vi "Script_Timing_Extract_Excit_Acq.vi"(7 "Script Text":string="script PireneaGas2sExcitAcq8s\n   wait until scriptTrigger0 \n   wait dd\n   generate AutLaserOn\n   wait 49000\n   generate AutLaserOnFilterOff\n   wait 1000\n   wait 600\n   generate AutLaserOnFilterOffTrapStart\n   wait 300\n   generate AutLaserOnFilterOffTrapStop\n   wait 2000\n   generate AutLaserOnFilterOn\n   wait 47100\n   generate AutLaserOff\n   wait 1950000\n   generate Gas1On\n   wait 150000\n   generate Gas1Off\n   wait 5850000\n   generate ExcitAcq\n   wait 1000000\n   generate FilterOff\n   wait 1000\n   generate FilterOffEmptyingStart\n   wait 1000000\n   generate FilterOffEmptyingStop\n   wait 2000\n   generate Zeros\nend script", 8 "error in (no error)":errorcluster, 9 "Script File":string="PireneaFree4sExcitAcq5s.txt", 10 "Script Path":path=path "D:/PIRENEA/TIMING_SCRIPTS") -> (0 "error out":errorcluster, 2 "Number of Excits":i16, 3 "Number of Acqs":i16)   [LabVIEW 2018]
uses:
  Global_Variables.vi
  <vilib>/regexp/Match Regular Expression.xnode
panel:
  out "Table of Excit":string[](array[string])
  out "Table of Acq":string[](array[string])
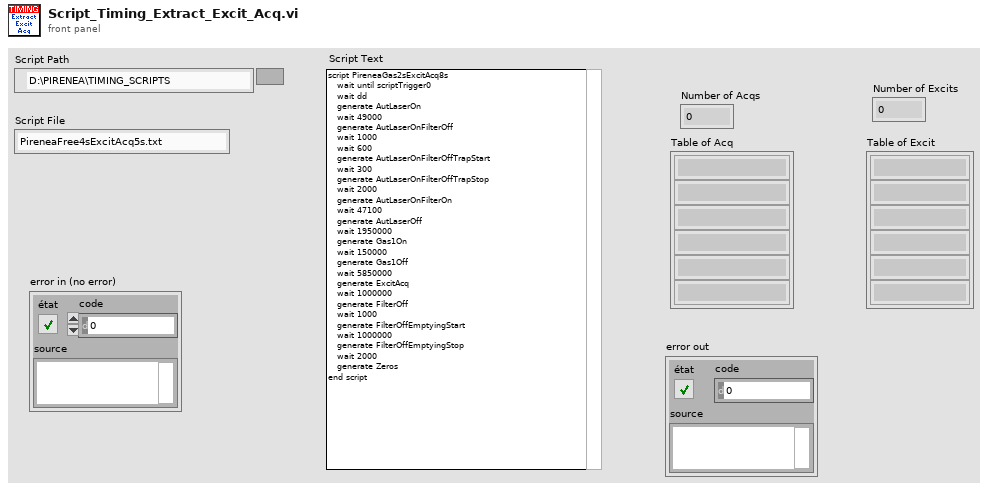
[diagram p1: front panel]
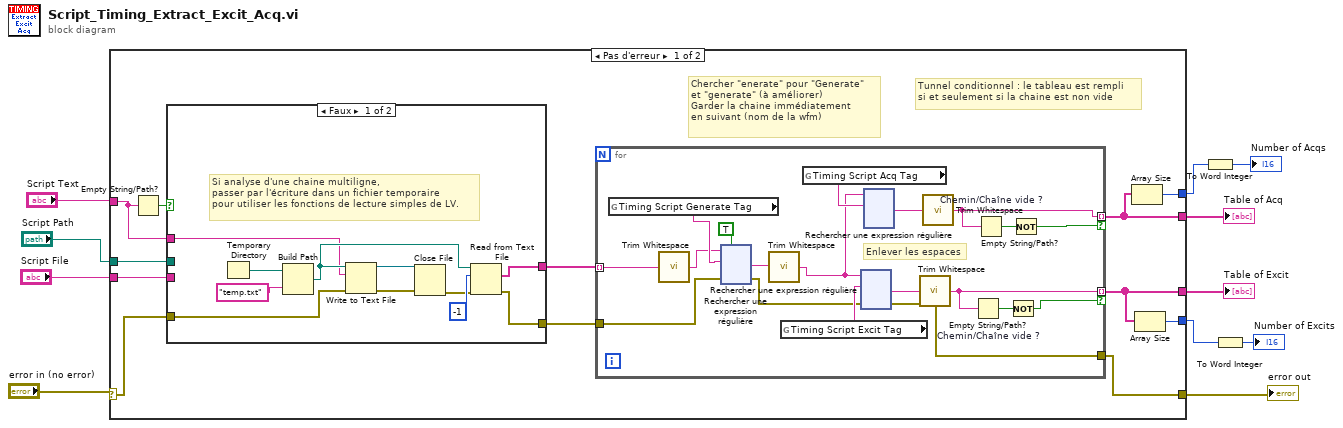
[diagram p0: block diagram]
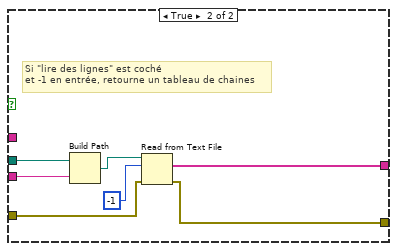
[diagram p2: hidden frame]
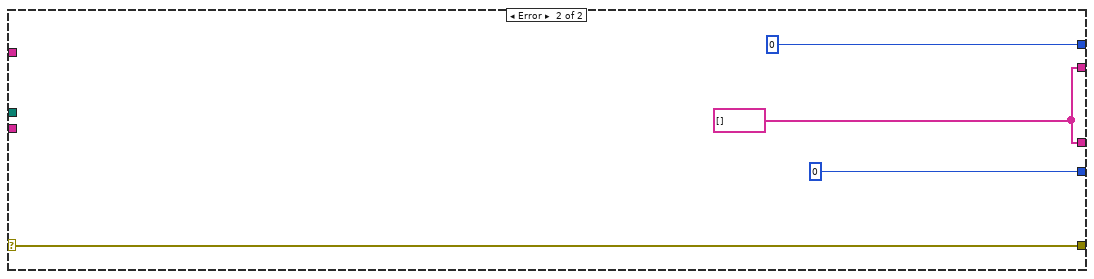
[diagram p3: hidden frame]
diagram:
  n1 = case shown="Pas d'erreur" "error in (no error)" {
    selector: "error in (no error)" -> [w14 w406]
    tunnel: "Script File" -> [w23 _]
    tunnel: [w12 w406] -> w9
    tunnel: "Script Path" -> [w22 _]
    tunnel: [w20 w405] -> w7
    tunnel: [w18 w405] -> w6
    tunnel: [w19 0] -> w5
    tunnel: [w17 0] -> w4
    tunnel: "Script Text" -> [w15 _]
    frame No Error {
      # "Tunnel conditionnel : le tableau est rempli\nsi et seulement si la chaine est non vide"
      # "Chercher \"enerate\" pour \"Generate\"\net \"generate\" (à améliorer)\nGarder la chaine immédiatement\nen suivant (nom de la wfm)"
      n2 = Empty String/Path?(string/path=w15) -> (empty?=w16:bool)
      n3 = case shown="Faux" w16 {
        tunnel: w23 -> [_ w41]
        tunnel: w22 -> [_ w40]
        tunnel: [w26 w37] -> w21
        tunnel: w15 -> [w27 _]
        tunnel: w14 -> [w25 w36]
        tunnel: [w24 w35] -> w13
        frame False {
          # "Si analyse d'une chaine multiligne,\npasser par l'écriture dans un fichier temporaire\npour utiliser les fonctions de lecture simples de LV."
          n4 = Temporary Directory() -> (w33:path)
          n5 = Build Path(base path=w33, name or relative path="temp.txt" ("nom ou chemin relatif")) -> (appended path=w30:path)
          n6 = Write to Text File(file (use dialog)=w30, text=w27, error in=w25) -> (refnum out=w31:refnum<file>, error out=w32:errorcluster)  [unwired: 1 in, 1 out]
          n7 = Close File(refnum=w31, error in=w32) -> (error out=w28:errorcluster)  [unwired: 1 out]
          n8 = Read from Text File(file (use dialog)=w30, count=-1 ("nombre"), error in=w28) -> (text=w26:string[], error out=w24:errorcluster)  [unwired: 1 in, 2 out]
        }
        frame True {
          # "Si \"lire des lignes\" est coché\net -1 en entrée, retourne un tableau de chaines"
          n9 = Build Path(base path=w40, name or relative path=w41) -> (appended path=w39:path)
          n10 = Read from Text File(file (use dialog)=w39, count=-1 ("nombre"), error in=w36) -> (text=w37:string[], error out=w35:errorcluster)  [unwired: 1 in, 2 out]
        }
      }
      n11 = for {
        tunnel: w21 -> [w60] mode=indexing
        tunnel: [w57] -> w20 mode=indexing if=w58
        tunnel: [w52] -> w18 mode=indexing if=w51
        tunnel: w13 -> [w45]
        tunnel: [w42] -> w12
        # "Enlever les espaces"
        n12 = global read "Global_Variables.vi" "Timing Script Generate Tag"() -> (w48:string)
        n13 = call <vilib>:"Trim Whitespace.vi"("string"=w60) -> ("trimmed string"=w47:string)  [unwired: 1 in]
        n14 = xnode "Rechercher une expression régulière"("chaîne en entrée"=w47, "expression régulière"=w48, "entrée d'erreur"=w45, "ignorer la casse ? (F)"=TRUE) -> ("après la correspondance"=w56:string, "sortie d'erreur"=w43:errorcluster)  [unwired: 2 in, 3 out]
        n15 = call <vilib>:"Trim Whitespace.vi"("string"=w56) -> ("trimmed string"=w44:string)  [unwired: 1 in]
        n16 = global read "Global_Variables.vi" "Timing Script Excit Tag"() -> (w50:string)
        n17 = global read "Global_Variables.vi" "Timing Script Acq Tag"() -> (w49:string)
        n18 = xnode "Rechercher une expression régulière"("chaîne en entrée"=w44, "expression régulière"=w50, "entrée d'erreur"=w43) -> ("toute l'expression"=w54:string, "sortie d'erreur"=w42:errorcluster)  [unwired: 3 in, 3 out]
        n19 = xnode "Rechercher une expression régulière"("chaîne en entrée"=w44, "expression régulière"=w49) -> ("toute l'expression"=w55:string)  [unwired: 4 in, 4 out]
        n20 = call <vilib>:"Trim Whitespace.vi"("string"=w54) -> ("trimmed string"=w52:string)  [unwired: 1 in]
        n21 = call <vilib>:"Trim Whitespace.vi"("string"=w55) -> ("trimmed string"=w57:string)  [unwired: 1 in]
        n22 = Empty String/Path? "Chemin/Chaîne vide ?"(string/path=w52) -> (empty?=w53:bool)
        n23 = Empty String/Path? "Chemin/Chaîne vide ?"(string/path=w57) -> (empty?=w59:bool)
        n24 = Not(x=w53) -> (.not. x?=w51:bool)
        n25 = Not(x=w59) -> (.not. x?=w58:bool)
      }
      n26 = Array Size(array=w20) -> (size(s)=w19:i32)
      n27 = Array Size(array=w18) -> (size(s)=w17:i32)
    }
    frame Error {
      w405 = string[] []
    }
  }
  "error out" <- w9
  "Table of Acq" <- w7
  "Table of Excit" <- w6
  n28 = To Word Integer(number=w5) -> (16bit integer=→"Number of Acqs":i16)
  n29 = To Word Integer(number=w4) -> (16bit integer=→"Number of Excits":i16)
